vi "Blink.vi"   [LabVIEW 2019]
uses:
  <vilib>/NI_Real-Time Target Support.lvlib
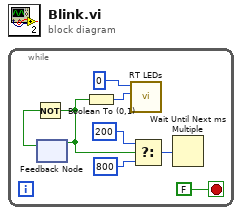
[diagram p0: block diagram]
diagram:
  n1 = while {
    stop <- FALSE stop-if-true
    n2 = feedback #1() -> (w6:bool)  [unwired: 1 in]
    n3 = Not(x=w6) -> (.not. x?=w5:bool)
    n4 = feedback-in #1(w5) -> ()
    n5 = Boolean To (0,1)(Boolean=w5) -> (0, 1=w4:i16)
    n6 = call <vilib>:"RT LEDs.vi"("State"=w4, "LED Num"=0) -> ()  [unwired: 4 in, 2 out]
    n7 = Select(t=u32 200 ("millisecond multiple"), s=w5, f=u32 800 ("millisecond multiple")) -> (s? t:f=w1:u32)
    n8 = Wait Until Next ms Multiple(millisecond multiple=w1) -> ()  [unwired: 1 out]
  }
